vi "GenerateMenu.vi"(8 "error in":errorcluster, 10 "menu ref in":refnum<k9>, 11 "SystemConfigRepo in":refnum<class "SystemConfigRepo.lvclass">) -> (0 "error out":errorcluster, 2 "menu ref out":refnum<k9>, 3 "SystemConfigRepo out":refnum<class "SystemConfigRepo.lvclass">)   [LabVIEW 2013, in "PL Framework Configuration Tool.lvlib" / "SystemConfigRepo.lvclass"]
uses:
  SystemConfigRepo.lvclass
  <vilib>/Utility/miscctls.llb/LVMenuShortCut.ctl
  <vilib>/NI/Configuration Framework/hierarchy repo/NISE_CEF_HierarchyRepo.lvclass
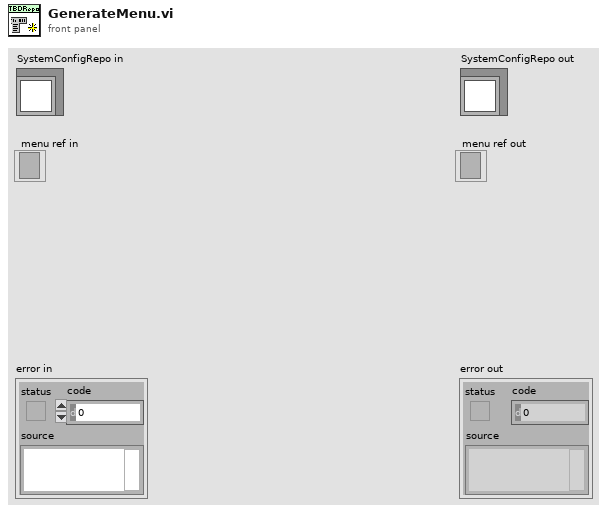
[diagram p1: front panel]
types:
  T1 = typedef "LVMenuShortCut.ctl" = cluster{"Include Shift Key?":bool, "Include Ctrl Key?":bool, "Shortcut Key":string}
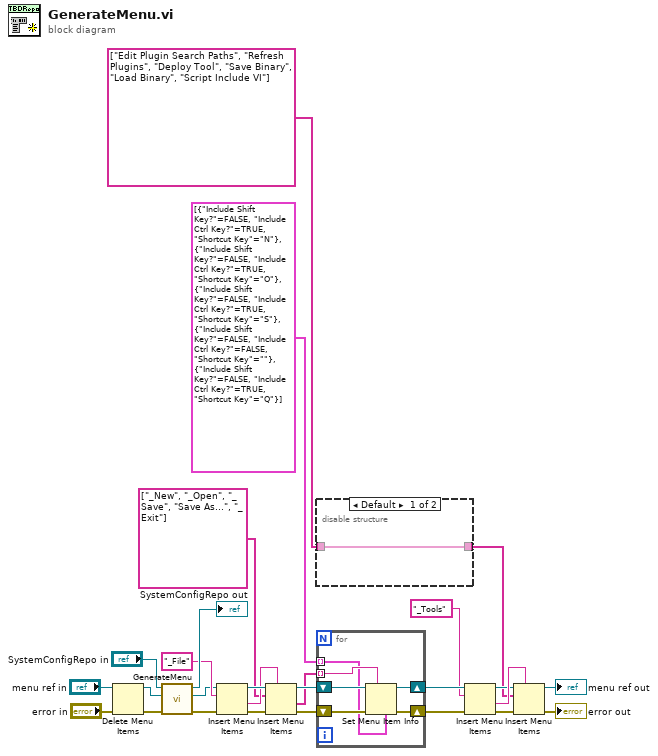
[diagram p0: block diagram]
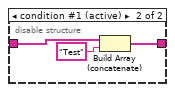
[diagram p2: hidden frame]
diagram:
  n1 = Delete Menu Items(6:"error in", 9:"menu ref in") -> (0:w7:errorcluster, 3:w5:refnum<k9>)  [unwired: 2 in]
  n2 = call-parent "GenerateMenu.vi"("error in"=w7, "menu ref in"=w5, "NISE_CEF_Repository in"="SystemConfigRepo in") -> ("error out"=w4:errorcluster, "menu ref out"=w3:refnum<k9>, "NISE_CEF_Repository out"=→"SystemConfigRepo out":refnum<class "SystemConfigRepo.lvclass">)  [unwired: 6 in]
  n3 = Insert Menu Items(6:w4, 8:"_File", 9:w3) -> (0:w21:errorcluster, 1:w22:string, 3:w23:refnum<k9>)  [unwired: 3 in]
  n4 = Insert Menu Items(5:w22, 6:w21, 8:string[] ["_New", "_Open", "_Save", "Save As...", "_Exit"] ("item names"), 9:w23) -> (0:w18:errorcluster, 1:w17:string[], 3:w19:refnum<k9>)  [unwired: 2 in]
  n5 = disable-structure shown="Default" {
    disable-tunnel: [w28 w30] -> w9
    disable-tunnel: string[] ["Edit Plugin Search Paths", "Refresh Plugins", "Deploy Tool", "Save Binary", "Load Binary", "Script Include VI"] ("item names") -> [w28 w31]
    frame condition #0 {
    }
    frame condition #1 (active) {
      n6 = Build Array (concatenate)(w31, "Test") -> (w30:string[])
    }
  }
  n7 = for {
    shift-right: [w35] -> w15
    shift-left: w19 -> [w37]
    tunnel: w17 -> [w34] mode=indexing
    tunnel: T1[] [{"Include Shift Key?"=FALSE, "Include Ctrl Key?"=TRUE, "Shortcut Key"="N"}, {"Include Shift Key?"=FALSE, "Include Ctrl Key?"=TRUE, "Shortcut Key"="O"}, {"Include Shift Key?"=FALSE, "Include Ctrl Key?"=TRUE, "Shortcut Key"="S"}, {"Include Shift Key?"=FALSE, "Include Ctrl Key?"=FALSE, "Shortcut Key"=""}, {"Include Shift Key?"=FALSE, "Include Ctrl Key?"=TRUE, "Shortcut Key"="Q"}] -> [w32] mode=indexing
    shift-right: [w33] -> w14
    shift-left: w18 -> [w36]
    n8 = Set Menu Item Info(4:w32, 7:w34, 8:w36, 11:w37) -> (0:w33:errorcluster, 3:w35:refnum<k9>)  [unwired: 3 in]
  }
  n9 = Insert Menu Items(6:w14, 8:"_Tools", 9:w15) -> (0:w12:errorcluster, 1:w13:string, 3:w11:refnum<k9>)  [unwired: 3 in]
  n10 = Insert Menu Items(5:w13, 6:w12, 8:w9, 9:w11) -> (0:→"error out":errorcluster, 3:→"menu ref out":refnum<k9>)  [unwired: 2 in, 1 out]
